vi "RT_Coriolis_Moment_in_DLR_Navigation_Reference_System_2(SubVI).vi"(0 "Data":dbl[][](array[numeric]), 5 "i":i32, 7 "Vehicle Parameters":T2, 11 "Rotation":T1) -> (4 "Mco (Nm)":dbl[](array[numeric]))   [LabVIEW 2017]
uses:
  <vilib>/Analysis/Matrix/Datatypes/RealMatrix.ctl
  <vilib>/Analysis/baseanly.llb/Real A x B.vi
  <vilib>/Analysis/Matrix/Numeric/Conversions/Array To Matrix - RA.vi
  <vilib>/Analysis/Matrix/Numeric/Conversions/Array To Matrix - RA2.vi
  <vilib>/Analysis/Matrix/Numeric/Conversions/Matrix To Array - RM.vi
  <vilib>/Analysis/NI_AALBase.lvlib
  <vilib>/Analysis/Matrix/NI_Matrix.lvlib
  <vilib>/Analysis/NI_AALPro.lvlib
panel:
  out "-I_p_matrix (kg.m^2/s)":T3
  out "OMEGA":dbl[](array[numeric])
  out "m":dbl
  out "Re":dbl[](array[numeric])
  out "re":dbl
  out "CoG (m)":dbl
  out "M_p (kg/s)":dbl
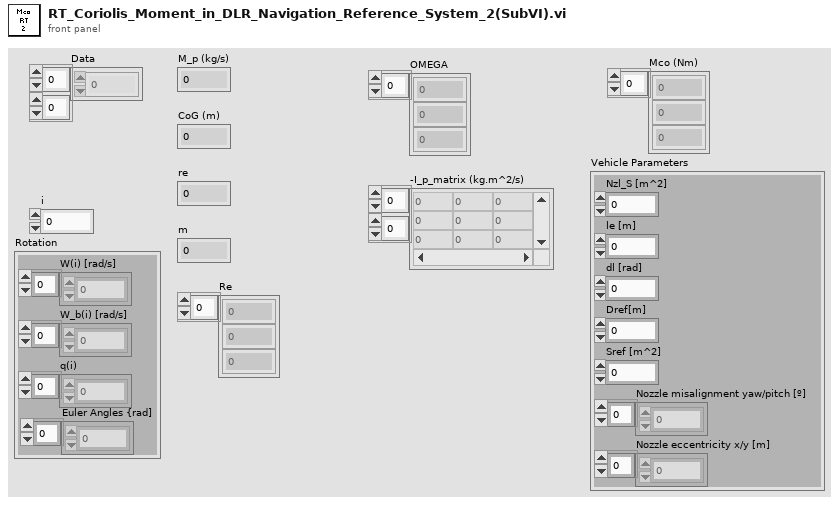
[diagram p1: front panel]
types:
  T1 = cluster{"W(i) [rad/s]":dbl[], "W_b(i) [rad/s]":dbl[], "q(i)":dbl[], "Euler Angles {rad]":dbl[]}
  T2 = cluster{"Nzl_S [m^2]":dbl, "le [m]":dbl, "dl [rad]":dbl, "Dref[m]":dbl, "Sref [m^2]":dbl, "Nozzle misalignment yaw/pitch [º]":dbl[], "Nozzle eccentricity x/y [m]":dbl[]}
  T3 = typedef "NI_Matrix.lvlib/RealMatrix.ctl" = dbl[][]
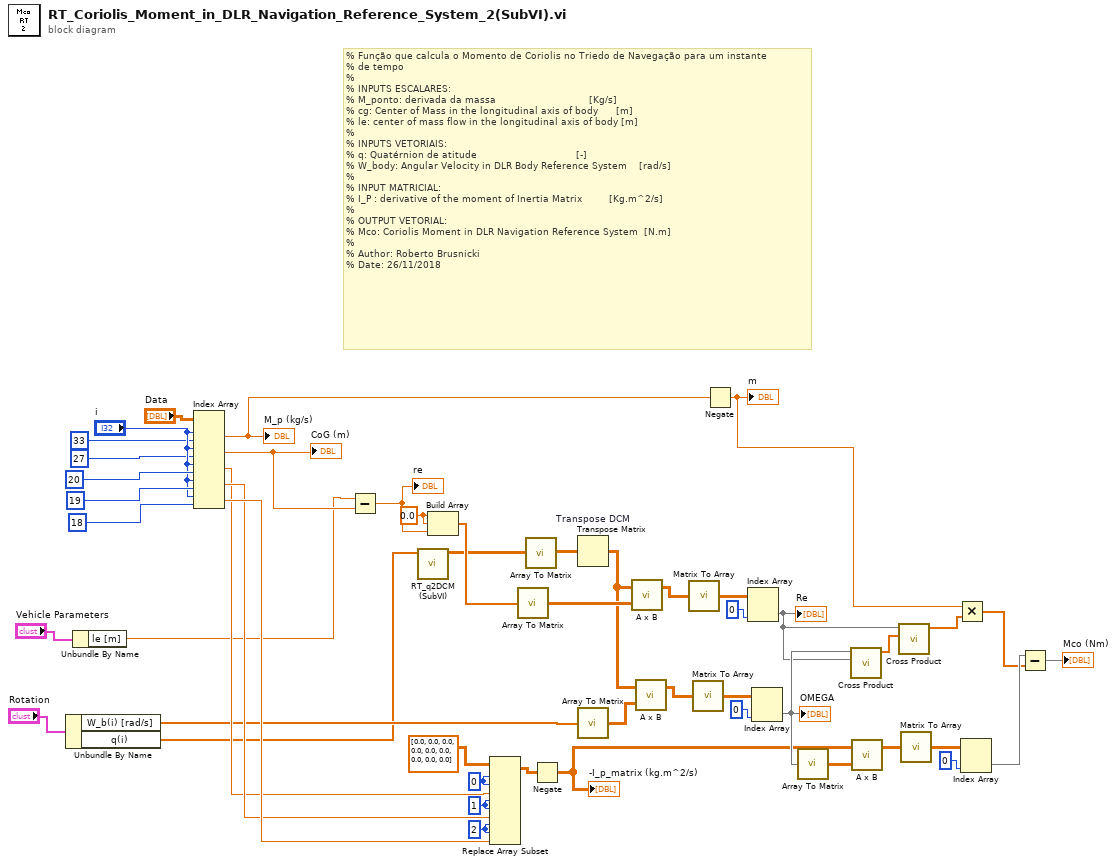
[diagram p0: block diagram]
diagram:
  w35 = 2 ("index (col)")
  w32 = 1 ("index (row)")
  w27 = 0 ("index (col)")
  w16 = 0.0 ("element")
  # "% Função que calcula o Momento de Coriolis no Triedo de Navegação para um instante\n% de tempo\n%\n% INPUTS ESCALARES:\n% M_ponto: derivada da massa                               [Kg/s]\n% cg: Center of Mass in the longitudinal axis of body      [m]\n% le: center of mass flow in the longitudinal axis of body [m]\n% \n% INPUTS VETORIAIS:\n% q: Quatérnion de atitude                                 [-]\n% W_body: Angular Velocity in DLR Body Reference System    [rad/s] \t\n%\n% INPUT MATRICIAL:\n% I_P : derivative of the moment of Inertia Matrix         [Kg.m^2/s]\n%\n% OUTPUT VETORIAL:\n% Mco: Coriolis Moment in DLR Navigation Reference System  [N.m]\n%\n% Author: Roberto Brusnicki\n% Date: 26/11/2018"
  n1 = Unbundle By Name("Rotation") -> ("W_b(i) [rad/s]"=w5:dbl[], "q(i)"=w3:dbl[])
  n2 = Unbundle By Name("Vehicle Parameters") -> ("le [m]"=w6:dbl)
  n3 = Index Array(array="Data", index (row) #1="i", index (col) #1=33 ("disabled index (col)"), index (row) #2="i", index (col) #2=27 ("disabled index (col)"), index (row) #3="i", index (col) #3=20 ("disabled index (col)"), index (row) #4="i", index (col) #4=19 ("disabled index (col)"), index (row) #5="i", index (col) #5=18 ("disabled index (col)")) -> (element #1=w13:dbl, element #2=w21:dbl, element #3=w31:dbl, element #4=w33:dbl, element #5=w34:dbl)
  "M_p (kg/s)" <- w13
  "CoG (m)" <- w21
  n4 = Subtract(x=w6, y=w21) -> (x-y=w17:dbl)
  "re" <- w17
  n5 = call "RT_q2DCM (SubVI).vi"("Quaternion"=w3) -> ("DCM"=w2:dbl[][])  [unwired: 10 in]
  n6 = Build Array(w16, w16, w17) -> (w15:dbl[])
  n7 = Replace Array Subset(array=T3 [[0.0, 0.0, 0.0], [0.0, 0.0, 0.0], [0.0, 0.0, 0.0]] ("transposed matrix"), new element #1=w31, index (row) #1=w27, index (col) #1=w27, new element #2=w33, index (row) #2=w32, index (col) #2=w32, new element #3=w34, index (row) #3=w35, index (col) #3=w35) -> (w37:T3)
  n8 = call-poly <vilib>:"Array To Matrix.vi"("Real 1D Array"=w15) -> ("Real Matrix (Column Vector)"=w18:T3)
  n9 = call-poly <vilib>:"Array To Matrix.vi"("Real 2D Array"=w2) -> ("Real Matrix"=w14:T3)
  n10 = Negate(x=w37) -> (-x=w38:T3)
  "-I_p_matrix (kg.m^2/s)" <- w38
  n11 = Transpose Matrix "Transpose DCM"(1:w14) -> (0:w10:T3)
  n12 = call-poly <vilib>:"Array To Matrix.vi"("Real 1D Array"=w5) -> ("Real Matrix (Column Vector)"=w12:T3)
  n13 = call-poly <vilib>:"A x B.vi"("B"=w18, "A"=w10) -> ("A x B"=w20:T3)  [unwired: 1 out]
  n14 = call-poly <vilib>:"A x B.vi"("B"=w12, "A"=w10) -> ("A x B"=w36:T3)  [unwired: 1 out]
  n15 = call-poly <vilib>:"Matrix To Array.vi"("Real Matrix"=w20) -> ("Real 2D Array"=w19:dbl[][])
  n16 = call-poly <vilib>:"Matrix To Array.vi"("Real Matrix"=w36) -> ("Real 2D Array"=w11:dbl[][])
  n17 = Negate(x=w13) -> (-x=w42:dbl)
  "m" <- w42
  n18 = Index Array(array=w19, index (col)=0 ("index (row)")) -> (element=w39:dbl[])  [unwired: 1 in]
  "Re" <- w39
  n19 = Index Array(array=w11, index (col)=0 ("index (row)")) -> (element=w44:dbl[])  [unwired: 1 in]
  "OMEGA" <- w44
  n20 = call-poly <vilib>:"Array To Matrix.vi"("Real 1D Array"=w44) -> ("Real Matrix (Column Vector)"=w45:T3)
  n21 = call <vilib>:"Cross Product.vi"("B Vector"=w39, "A Vector"=w44) -> ("Cross Product"=w40:dbl[])  [unwired: 8 in, 1 out]
  n22 = call-poly <vilib>:"A x B.vi"("B"=w45, "A"=w38) -> ("A x B"=w43:T3)  [unwired: 1 out]
  n23 = call <vilib>:"Cross Product.vi"("B Vector"=w40, "A Vector"=w39) -> ("Cross Product"=w41:dbl[])  [unwired: 8 in, 1 out]
  n24 = call-poly <vilib>:"Matrix To Array.vi"("Real Matrix"=w43) -> ("Real 2D Array"=w46:dbl[][])
  n25 = Multiply(x=w42, y=w41) -> (x*y=w47:dbl[])
  n26 = Index Array(array=w46, index (col)=0 ("index (row)")) -> (element=w48:dbl[])  [unwired: 1 in]
  n27 = Subtract(x=w48, y=w47) -> (x-y=→"Mco (Nm)":dbl[])
